vi "GEA2 Message to LEUI_LEDs.vi"(5 "Ignore Brightness":bool, 7 "Raw Data In":string) -> (8 "LEUI_LEDs":T1)   [LabVIEW 2016, in "TL27.lvlib"]
uses:
  Projects/TL27.lvlib
  controls/LEUI_LEDs.ctl
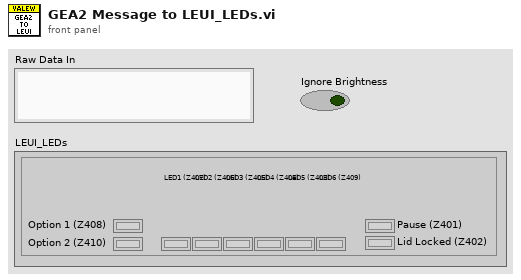
[diagram p1: front panel]
types:
  T1 = typedef "TL27.lvlib/LEUI_LEDs.ctl" = cluster{"Pause (Z401)":bool, "Lid Locked (Z402)":bool, "LED1 (Z407)":bool, "LED2 (Z406)":bool, "LED3 (Z405)":bool, "LED4 (Z404)":bool, "LED5 (Z403)":bool, "LED6 (Z409)":bool, "Option 1 (Z408)":bool, "Option 2 (Z410)":bool}
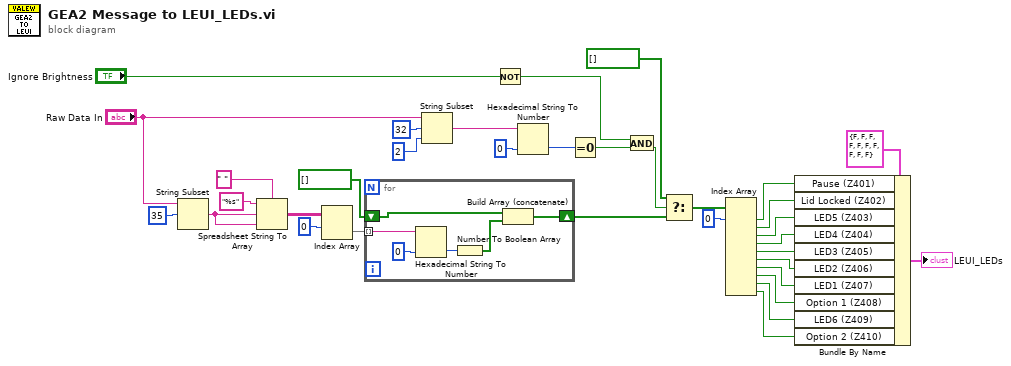
[diagram p0: block diagram]
diagram:
  n1 = String Subset(string="Raw Data In", offset (0)=35) -> (substring=w27:string)  [unwired: 1 in]
  n2 = Spreadsheet String To Array(delimiter (Tab)=" ", format string="%s", spreadsheet string=w27, array type (2D Dbl)=w27) -> (array=w31:string[][])
  n3 = Index Array(array=w31, index (row)=0) -> (element=w28:string[])  [unwired: 1 in]
  n4 = for {
    tunnel: w28 -> [w40] mode=indexing
    shift-right: [w36] -> w20
    shift-left: bool[] [] -> [w38]
    n5 = Hexadecimal String To Number(string=w40, default (0uL)=u8 0) -> (number=w39:u8)  [unwired: 1 in, 1 out]
    n6 = Number To Boolean Array(number=w39) -> (Boolean array=w37:bool[])
    n7 = Build Array (concatenate)(w38, w37) -> (w36:bool[])
  }
  n8 = String Subset(string="Raw Data In", offset (0)=32, length (rest)=2 ("length (rest)")) -> (substring=w24:string)
  n9 = Not(x="Ignore Brightness") -> (.not. x?=w1:bool)
  n10 = Hexadecimal String To Number(string=w24, default (0uL)=u32 0 ("default (0 U32)")) -> (number=w22:u32)  [unwired: 1 in, 1 out]
  n11 = Equal To 0?(x=w22) -> (x = 0?=w21:bool)
  n12 = And(x=w1, y=w21) -> (x .and. y?=w3:bool)
  n13 = Select(t=bool[] [], s=w3, f=w20) -> (s? t:f=w18:bool[])
  n14 = Index Array(array=w18, index #1=0 ("index")) -> (element #1=w17:bool, element #2=w9:bool, element #3=w14:bool, element #4=w13:bool, element #5=w12:bool, element #6=w11:bool, element #7=w10:bool, element #8=w6:bool, element #9=w5:bool, element #10=w4:bool)  [unwired: 9 in]
  n15 = Bundle By Name(cluster=T1 {"Pause (Z401)"=FALSE, "Lid Locked (Z402)"=FALSE, "LED1 (Z407)"=FALSE, "LED2 (Z406)"=FALSE, "LED3 (Z405)"=FALSE, "LED4 (Z404)"=FALSE, "LED5 (Z403)"=FALSE, "LED6 (Z409)"=FALSE, "Option 1 (Z408)"=FALSE, "Option 2 (Z410)"=FALSE} ("LEUI_LEDs"), "Pause (Z401)"=w17, "Lid Locked (Z402)"=w9, "LED5 (Z403)"=w14, "LED4 (Z404)"=w13, "LED3 (Z405)"=w12, "LED2 (Z406)"=w11, "LED1 (Z407)"=w10, "Option 1 (Z408)"=w6, "LED6 (Z409)"=w5, "Option 2 (Z410)"=w4) -> (→"LEUI_LEDs":T1)
